vi "Update Scrollbars.vi"(8 "error in (no error)":errorcluster, 11 "2DArrayManager in":refnum<class "2DArrayManager.lvclass">) -> (0 "error out":errorcluster, 3 "2DArrayManager out":refnum<class "2DArrayManager.lvclass">)   [LabVIEW 2020, in "OOPanel.lvlib" / "2DArrayManager.lvclass"]
uses:
  2DArrayManager.lvclass
  2DArrayManager.lvclass/2DArrayManager.ctl
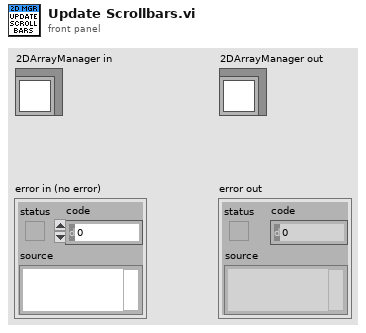
[diagram p1: front panel]
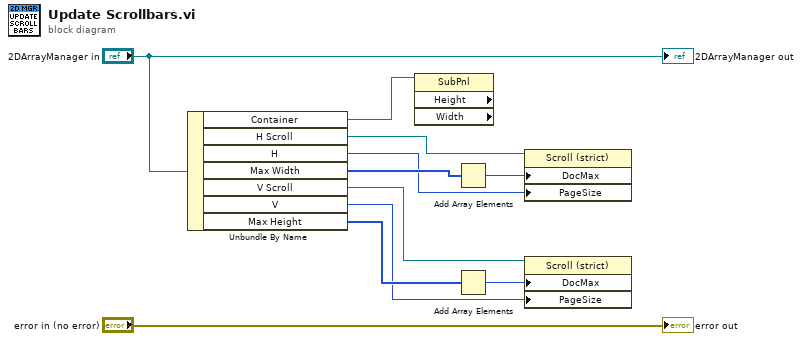
[diagram p0: block diagram]
diagram:
  n1 = Unbundle By Name("2DArrayManager in") -> ("Container"=w7:refnum<vi>, "H Scroll"=w6:refnum<vi>, "H"=w1:i32, "Max Width"=w2:u32[], "V Scroll"=w8:refnum<vi>, "V"=w5:i32, "Max Height"=w9:u32[])
  n2 = property class="SubPnl" props=["Height", "Width"](reference=w7) -> ()  [unwired: 1 in, 4 out]
  n3 = Add Array Elements(numeric array=w2) -> (sum=w3:u32)
  n4 = Add Array Elements(numeric array=w9) -> (sum=w4:u32)
  n5 = property class="Scroll (strict)"(reference=w6, "DocMax"=w3, "PageSize"=w1) -> ()  [unwired: 1 in, 2 out]
  n6 = property class="Scroll (strict)"(reference=w8, "DocMax"=w4, "PageSize"=w5) -> ()  [unwired: 1 in, 2 out]
  "error out" <- "error in (no error)"
  "2DArrayManager out" <- "2DArrayManager in"
